vi "Write UTF-8 String.vi"(8 "error in (no error)":errorcluster, 10 "UTF-8 String":string, 11 "UTF-8 String in":refnum<class "UTF-8 String.lvclass">) -> (0 "error out":errorcluster, 3 "UTF-8 String out":refnum<class "UTF-8 String.lvclass">)   [LabVIEW 2010, in "JKI Unicode.lvlib" / "UTF-8 String.lvclass"]
uses:
  UTF-8 String.lvclass
  Byte Stream.ctl
  UTF-8 String.lvclass/UTF-8 String.ctl
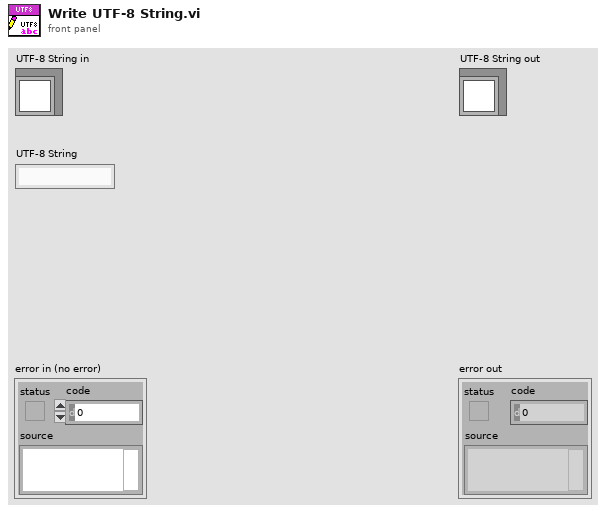
[diagram p1: front panel]
types:
  T1 = typedef "JKI Unicode.lvlib/UTF-8 String.lvclass/Byte Stream.ctl" = u8[]
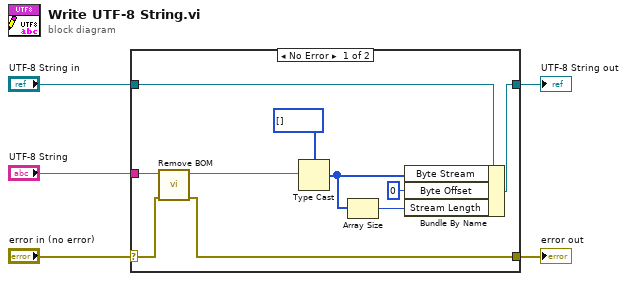
[diagram p0: block diagram]
diagram:
  n1 = case shown="No Error" "error in (no error)" {
    selector: "error in (no error)" -> [w8 w16]
    tunnel: [w7 w16] -> w4
    tunnel: [w14 w17] -> w2
    tunnel: "UTF-8 String in" -> [w15 w17]
    tunnel: "UTF-8 String" -> [w9 _]
    frame No Error {
      n2 = call "Remove BOM.vi"("error in (no error)"=w8, "String in"=w9) -> ("error out"=w7:errorcluster, "String out"=w6:string)  [unwired: 8 in]
      n3 = Type Cast(type=T1 [] ("Byte Stream"), x=w6) -> (*(type *) &x=w10:T1)
      n4 = Array Size(array=w10) -> (size(s)=w11:i32)
      n5 = Bundle By Name(cluster=w15, "Byte Stream"=w10, "Byte Offset"=0 ("Offset"), "Stream Length"=w11) -> (w14:refnum<class "UTF-8 String.lvclass">)
    }
    frame Error {
    }
  }
  "error out" <- w4
  "UTF-8 String out" <- w2
